vi "UE9 Single Pulse Output (no-timer).vi"() -> ()   [LabVIEW 2021]
panel:
  in  "USB Connection Type":bool=TRUE
  in  "Digital I/O Channel":i32
  in  "Pulse Time (milliseconds)":i32=100
  out "Error Message":string
  out "error out":errorcluster
  # "Uses a software delay to create a single positive pulse on a digital output line on the UE9."
  # "0-7       FIO0-FIO7\n8-15     EIO0-EIO7\n16-19   CIO0-CIO3"
  # "USB High-High\n\nUSB Other"
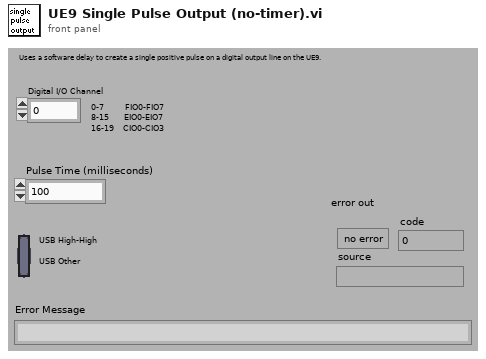
[diagram p1: front panel]
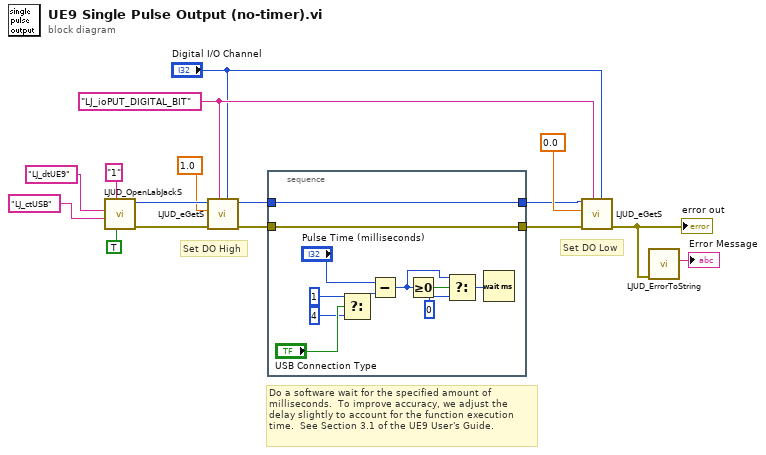
[diagram p0: block diagram]
diagram:
  w5 = "LJ_ioPUT_DIGITAL_BIT" ("IOType")
  # "Do a software wait for the specified amount of\nmilliseconds.  To improve accuracy, we adjust the\ndelay slightly to account for the function execution\ntime.  See Section 3.1 of the UE9 User's Guide."
  # "Set DO Low"
  # "Set DO High"
  n1 = call "LJUD_OpenLabJackS.vi"("FirstFound"=TRUE, "Address"="1", "ConnectionType"="LJ_ctUSB", "DeviceType"="LJ_dtUE9") -> ("error out"=w10:errorcluster, "Handle"=w11:i32)  [unwired: 5 in, 1 out]
  n2 = call "LJUD_eGetS.vi"("Channel"="Digital I/O Channel", "IOType"=w5, "error in"=w10, "Value Write"=1.0, "Handle In"=w11) -> ("error out"=w8:errorcluster, "Handle Out"=w2:i32)  [unwired: 4 in, 1 out]
  n3 = stacked-sequence {
    tunnel: w8 -> [w27]
    tunnel: [w27] -> w7
    tunnel: w2 -> [w24]
    tunnel: [w24] -> w1
    frame #0 {
      n4 = Select(t=1, s="USB Connection Type", f=4) -> (s? t:f=w21:i32)
      n5 = Subtract(x="Pulse Time (milliseconds)", y=w21) -> (x-y=w19:i32)
      n6 = Greater Or Equal To 0?(x=w19) -> (x >= 0?=w20:bool)
      n7 = Select(t=w19, s=w20, f=0 ("lower limit")) -> (s? t:f=w17:i32)
      n8 = Wait (ms)(milliseconds to wait=w17) -> ()  [unwired: 1 out]
    }
  }
  n9 = call "LJUD_eGetS.vi"("Channel"="Digital I/O Channel", "IOType"=w5, "error in"=w7, "Value Write"=0.0, "Handle In"=w1) -> ("error out"=w6:errorcluster)  [unwired: 4 in, 2 out]
  "error out" <- w6
  n10 = call "LJUD_ErrorToString.vi"("error in"=w6) -> ("String"=→"Error Message":string)  [unwired: 10 in]
